vi "Print Error.vi"(5 "Custom Device? (T)":bool=TRUE, 7 "error out":errorcluster, 9 "Note (empty)":string, 10 "Your code's public name":string) -> ()   [LabVIEW 2010, in "Flight Gear Data Custom Device.lvlib"]
doc: "Prints error information out to the console. Provide your code's public name. For example, if your code is about J1939, put that here so the user knows what this printed error information has to do with.\n\nIf this is not a NI VeriStand custom device, write false to the Custom Device? input. This will change the error output and cause this to ignore error -2206.\n\nIf the 'note' field is empty, it is not printed to the console.\n\nExample output 1:\n******J1939 ERROR******\nSource: blah.vi\nCode: 535\n******J1939 ERROR******\n\nExample output 2:\n******XCP and CCP Master CUSTOM DEVICE ERROR******\nSource: blah.vi\nCode: 535\nUser Note: before write\n******XCP and CCP Master CUSTOM DEVICE ERROR******"
uses:
  Flight Gear Data Custom Device.lvlib
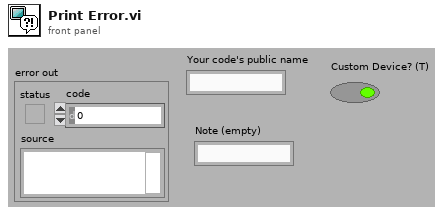
[diagram p1: front panel]
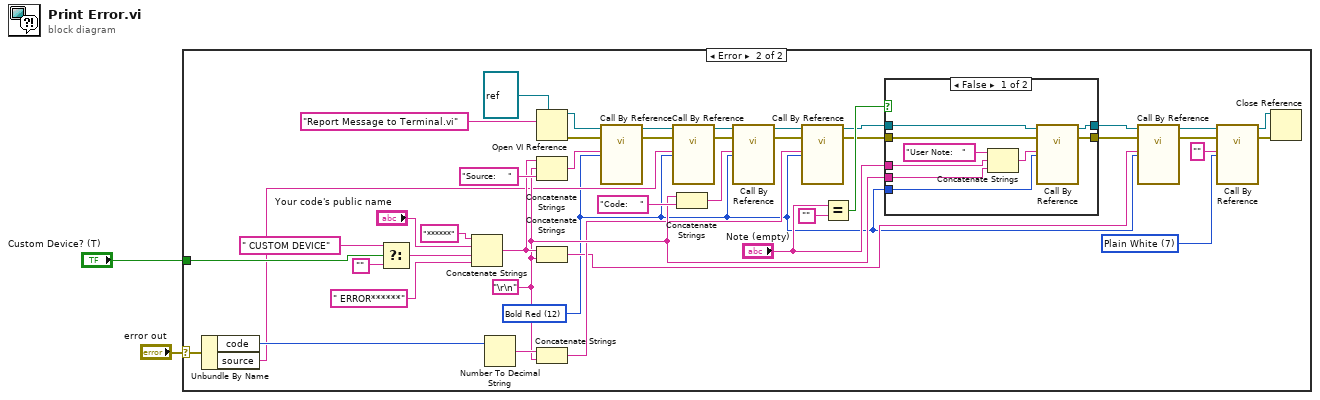
[diagram p0: block diagram]
diagram:
  n1 = case shown="Error" "error out" {
    selector: "error out" -> [_ w45]
    tunnel: "Custom Device? (T)" -> [_ w29]
    frame No Error {
    }
    frame Error {
      w24 = u16 7 items=["Plain White"=7, "Bold White"=15, "Bold Blue"=9, "Bold Green"=10, "Bold Red"=12] ("Color (Plain White)")
      w4 = u16 12 items=["Plain White"=7, "Bold White"=15, "Bold Blue"=9, "Bold Green"=10, "Bold Red"=12] ("Color (Plain White)")
      w32 = "\r\n"
      n2 = Unbundle By Name(w45) -> ("code"=w44:i32, "source"=w21:string)
      n3 = Select(t=" CUSTOM DEVICE" ("String"), s=w29, f="") -> (s? t:f=w30:string)
      n4 = Concatenate Strings("******" ("String"), "Your code's public name", w30, " ERROR******" ("String")) -> (w36:string)
      n5 = Number To Decimal String(number=w44) -> (decimal integer string=w41:string)  [unwired: 1 in]
      n6 = Open VI Reference(type specifier VI Refnum (for type only)=refnum<vi> refnum, vi path="Report Message to Terminal.vi") -> (vi reference=w19:refnum<vi>, error out=w18:errorcluster)  [unwired: 1 in, 3 out]
      n7 = Concatenate Strings(w36, w32, "Source:    " ("String")) -> (w23:string)
      n8 = Concatenate Strings(w36, w32) -> (w5:string)
      n9 = Concatenate Strings(w41, w32) -> (w14:string)
      n10 = call-by-ref "?"(reference=w19, error in=w18, "Color (Plain White)"=w4, "Message"=w23) -> (reference out=w20:refnum<vi>, error out=w22:errorcluster)  [unwired: 9 in, 1 out]
      n11 = call-by-ref "?"(reference=w20, error in=w22, "Color (Plain White)"=w4, "Message"=w21) -> (reference out=w15:refnum<vi>, error out=w16:errorcluster)  [unwired: 9 in, 1 out]
      n12 = Concatenate Strings(w32, "Code:    " ("String")) -> (w17:string)
      n13 = call-by-ref "?"(reference=w15, error in=w16, "Color (Plain White)"=w4, "Message"=w17) -> (reference out=w13:refnum<vi>, error out=w12:errorcluster)  [unwired: 9 in, 1 out]
      n14 = call-by-ref "?"(reference=w13, error in=w12, "Color (Plain White)"=w4, "Message"=w14) -> (reference out=w10:refnum<vi>, error out=w11:errorcluster)  [unwired: 9 in, 1 out]
      n15 = Equal?(x="Note (empty)", y="") -> (x = y?=w34:bool)
      n16 = case shown="False" w34 {
        tunnel: "Note (empty)" -> [w53 _]
        tunnel: w32 -> [w52 _]
        tunnel: [w49 w56] -> w9
        tunnel: w11 -> [w51 w56]
        tunnel: w10 -> [w48 w55]
        tunnel: [w47 w55] -> w6
        tunnel: w4 -> [w46 _]
        frame False {
          n17 = Concatenate Strings("User Note:   " ("string"), w53, w52) -> (w50:string)
          n18 = call-by-ref "?"(reference=w48, error in=w51, "Color (Plain White)"=w46, "Message"=w50) -> (reference out=w47:refnum<vi>, error out=w49:errorcluster)  [unwired: 9 in, 1 out]
        }
        frame True {
        }
      }
      n19 = call-by-ref "?"(reference=w6, error in=w9, "Color (Plain White)"=w4, "Message"=w5) -> (reference out=w7:refnum<vi>, error out=w8:errorcluster)  [unwired: 9 in, 1 out]
      n20 = call-by-ref "?"(reference=w7, error in=w8, "Color (Plain White)"=w24, "Message"="") -> (reference out=w25:refnum<vi>, error out=w26:errorcluster)  [unwired: 9 in, 1 out]
      n21 = Close Reference(reference=w25, error in (no error)=w26) -> ()  [unwired: 1 out]
    }
  }
